vi "Launch Subordinates.vi"(8 "error in":errorcluster, 11 "Base Software in":refnum<class "Main.lvclass">) -> (0 "error out":errorcluster, 3 "Base Software out":refnum<class "Main.lvclass">)   [LabVIEW 2023, in "Main.lvlib" / "Main.lvclass"]
doc: "This routine launches the main Actor Components:\n\n1. <b>Fault Monitor</b>\n2. <b>Debugger</b>\n3. <b>Configuration UI</b>\n4. <b>Chronometer</b>\n5. <b>Manual UI</b>\n6. <b>Manual Buttons</b>\n7. <b>Report Generator</b>\n8. <b>Report Viewer</b>"
uses:
  Project/Main.lvclass
  builds/Engine/Engine.lvlibp/Project/Engine.lvclass
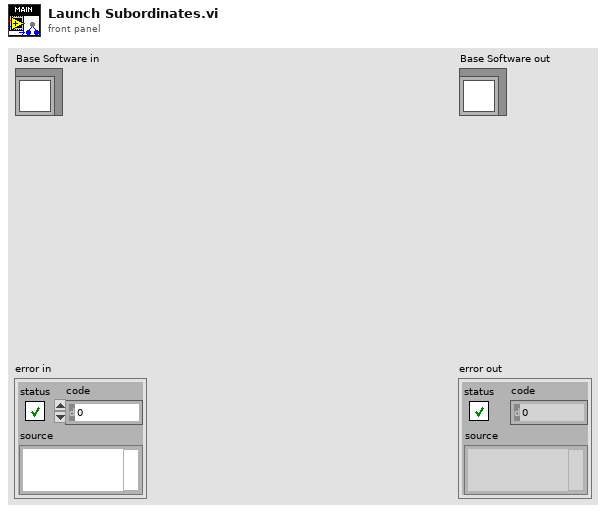
[diagram p1: front panel]
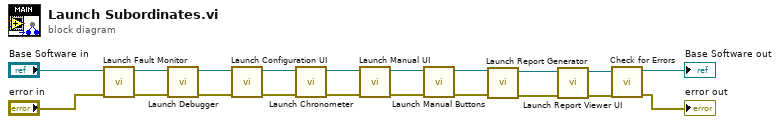
[diagram p0: block diagram]
diagram:
  n1 = call "Launch Fault Monitor.vi"("error in"="error in", "Base Software in"="Base Software in") -> ("error out"=w17:errorcluster, "Base Software out"=w19:refnum<class "Main.lvclass">)  [unwired: 8 in]
  n2 = call "Launch Debugger.vi"("error in"=w17, "Base Software in"=w19) -> ("error out"=w16:errorcluster, "Base Software out"=w20:refnum<class "Main.lvclass">)  [unwired: 8 in]
  n3 = call "Launch Configuration UI.vi"("error in"=w16, "Base Software in"=w20) -> ("error out"=w11:errorcluster, "Base Software out"=w12:refnum<class "Main.lvclass">)  [unwired: 8 in]
  n4 = call "Launch Chronometer.vi"("error in"=w11, "Base Software in"=w12) -> ("error out"=w9:errorcluster, "Base Software out"=w10:refnum<class "Main.lvclass">)  [unwired: 8 in]
  n5 = call "Launch Manual UI.vi"("error in"=w9, "Base Software in"=w10) -> ("error out"=w7:errorcluster, "Base Software out"=w8:refnum<class "Main.lvclass">)  [unwired: 8 in]
  n6 = call "Launch Manual Buttons.vi"("error in"=w7, "Base Software in"=w8) -> ("error out"=w6:errorcluster, "Base Software out"=w5:refnum<class "Main.lvclass">)  [unwired: 8 in]
  n7 = call "Launch Report Generator.vi"("error in"=w6, "Base Software in"=w5) -> ("error out"=w3:errorcluster, "Base Software out"=w4:refnum<class "Main.lvclass">)  [unwired: 8 in]
  n8 = call "Launch Report Viewer UI.vi"("error in"=w3, "Base Software in"=w4) -> ("error out"=w1:errorcluster, "Base Software out"=w2:refnum<class "Main.lvclass">)  [unwired: 8 in]
  n9 = call "Check for Errors.vi"("error in"=w1, "Engine in"=w2) -> ("error out"=→"error out":errorcluster, "Engine out"=→"Base Software out":refnum<class "Main.lvclass">)  [unwired: 8 in]
